vi "Handle State.vi"(8 "error in (no error)":errorcluster, 9 "Sender":refnum<class "Message Enqueuer.lvclass">, 10 "Process State":T1, 11 "CoolApp in":refnum<class "CoolApp.lvclass">) -> (0 "error out":errorcluster, 3 "CoolApp out":refnum<class "CoolApp.lvclass">)   [LabVIEW 2020, in "LAF2024Q2.lvlib" / "CoolApp.lvclass"]
uses:
  CoolApp.lvclass
  C:/dev/lv20CE/laf-2024-q2/LAF2024Q2/CoolAppProcess/CoolAppProcess.lvclass
  Process State.ctl
  <vilib>/ActorFramework/Message Enqueuer/Message Enqueuer.lvclass
  State Update.ctl
  Nested.ctl
  CoolApp.lvclass/CoolApp.ctl
  LAF2024Q2.lvlib
  CoolAppProcess/CoolAppProcess.lvclass
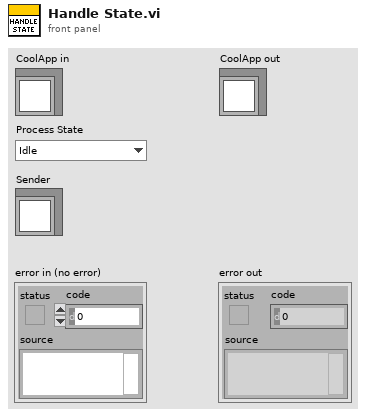
[diagram p1: front panel]
types:
  T1 = typedef "LAF2024Q2.lvlib/Process State.ctl" = enum16{"Idle", "Initializing", "Starting", "Running", "Stopping", "Stopped"}
  T2 = typedef "LAF2024Q2.lvlib/CoolApp.lvclass/State Update.ctl" = cluster{"Nested":T3, "Process State":T1}
  T3 = typedef "LAF2024Q2.lvlib/CoolApp.lvclass/Nested.ctl" = enum16{"DAQ", "Chart"}
  T4 = map{refnum<class "Message Enqueuer.lvclass">, T3}
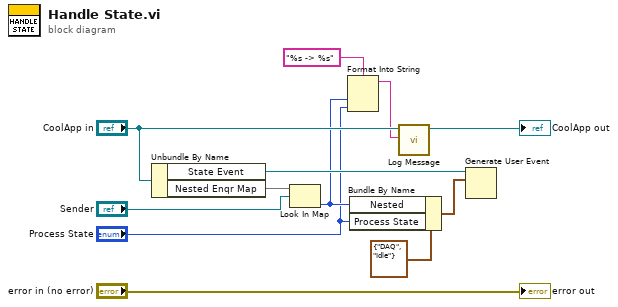
[diagram p0: block diagram]
diagram:
  n1 = Unbundle By Name("CoolApp in") -> ("State Event"=w8:refnum<user-event>, "Nested Enqr Map"=w10:T4)
  n2 = Look In Map(map=w10, key="Sender") -> (value=w3:T3)  [unwired: 1 in, 1 out]
  n3 = Format Into String(format string="%s -> %s", w3, "Process State") -> (resulting string=w1:string)  [unwired: 2 in, 1 out]
  n4 = Bundle By Name(cluster=T2 {"Nested"=enum."DAQ", "Process State"=enum."Idle"} ("State Update"), "Nested"=w3, "Process State"="Process State") -> (w6:T2)
  n5 = call "Log Message.vi"("Message"=w1, "CoolAppProcess in"="CoolApp in") -> ("CoolAppProcess out"=→"CoolApp out":refnum<class "CoolApp.lvclass">)  [unwired: 8 in, 1 out]
  n6 = Generate User Event(user event=w8, event data cluster=w6) -> ()  [unwired: 2 in, 2 out]
  "error out" <- "error in (no error)"
